vi "init Tests.vi"(8 "error in (no error)":errorcluster caption="Error in", 11 "Class 4 Eingang":refnum<class "Class 4.lvclass"> caption="DNL_LabVIEW Object in") -> (0 "error out":errorcluster caption="Error out", 3 "Class 4 Ausgang":refnum<class "Class 4.lvclass"> caption="DNL_LabVIEW Object out")   [LabVIEW 2013, in "Class 4.lvclass"]
doc: "Initilisiert die Standard-Tests für das Entsprechende Gerät"
uses:
  Class 4.lvclass
  Tests/TestTest/TestTest.lvclass
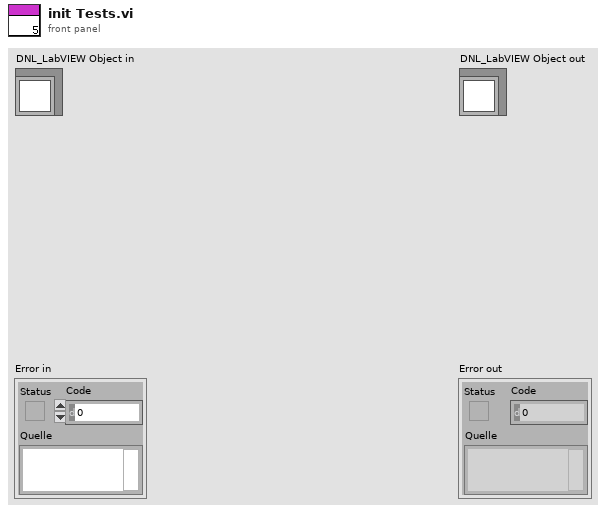
[diagram p1: front panel]
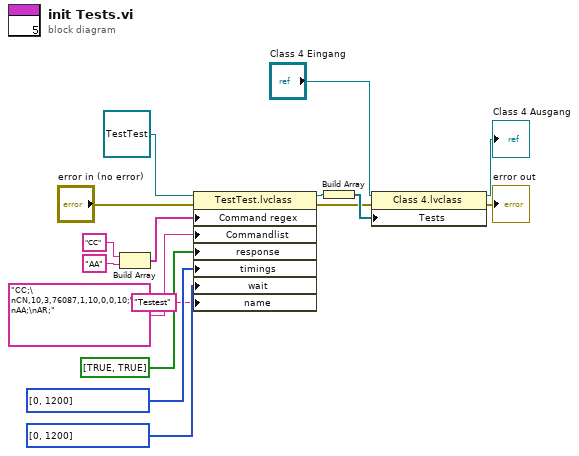
[diagram p0: block diagram]
diagram:
  n1 = Build Array("CC", "AA") -> (w14:string[])
  n2 = property class="TestTest.lvclass"(reference=refnum<class "TestTest.lvclass"> refnum ("TestTest.lvclass"), error in="error in (no error)", "Command regex"=w14, "Commandlist"="CC;\nCN,10,3,76087,1,10,0,0,10;\nAA;\nAR;", "response"=bool[] [TRUE, TRUE], "timings"=i32[] [0, 1200], "wait"=u32[] [0, 1200], "name"="Testest") -> (reference out=w11:refnum<class "TestTest.lvclass">, error out=w7:errorcluster)
  n3 = Build Array(w11) -> (w10:refnum<class "TestTest.lvclass">[])
  n4 = property class="Class 4.lvclass"(reference="Class 4 Eingang", error in=w7, "Tests"=w10) -> (reference out=→"Class 4 Ausgang":refnum<class "Class 4.lvclass">, error out=→"error out":errorcluster)
